vi "MTS_GenGridScanList.vi"(8 "Offsets":dbl[](array[numeric]), 9 "Points":u16[](array[numeric]), 11 "Starting":dbl[](array[numeric])) -> (0 "Grid Points":dbl[][](array[numeric]))   [LabVIEW 2011]
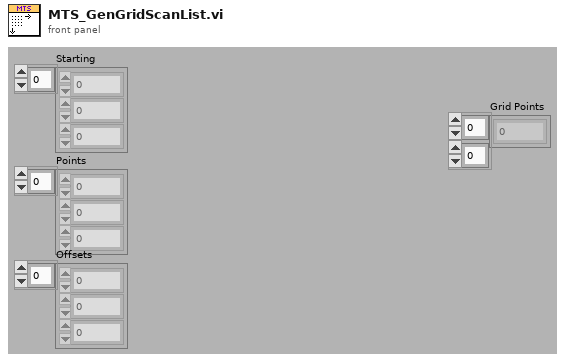
[diagram p1: front panel]
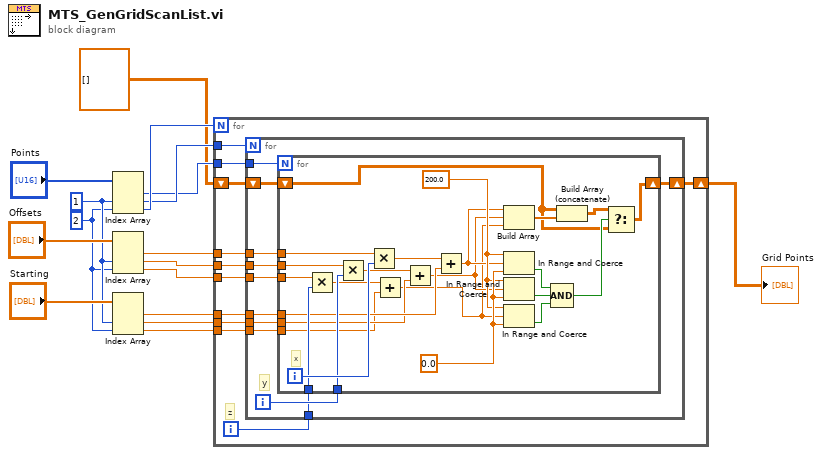
[diagram p0: block diagram]
diagram:
  w12 = 2 ("index")
  w13 = 1 ("index")
  n1 = Index Array(array="Points", index #2=w13, index #3=w12) -> (element #1=w9:u16, element #2=w10:u16, element #3=w11:u16)  [unwired: 1 in]
  n2 = Index Array(array="Offsets", index #2=w13, index #3=w12) -> (element #1=w5:dbl, element #2=w4:dbl, element #3=w3:dbl)  [unwired: 1 in]
  n3 = Index Array(array="Starting", index #2=w13, index #3=w12) -> (element #1=w8:dbl, element #2=w7:dbl, element #3=w6:dbl)  [unwired: 1 in]
  n4 = for {
    N: w11 -> [_]
    tunnel: w10 -> [w27]
    tunnel: w9 -> [w26]
    tunnel: w8 -> [w25]
    tunnel: w7 -> [w24]
    tunnel: w6 -> [w23]
    tunnel: w5 -> [w22]
    tunnel: w4 -> [w21]
    tunnel: w3 -> [w20]
    shift-right: [w17] -> w1
    shift-left: dbl[][] [] ("Grid Points") -> [w18]
    i -> [w19]
    # "z"
    n5 = for {
      N: w27 -> [_]
      tunnel: w26 -> [w38]
      tunnel: w25 -> [w37]
      tunnel: w24 -> [w36]
      tunnel: w23 -> [w35]
      tunnel: w22 -> [w34]
      tunnel: w21 -> [w33]
      tunnel: w20 -> [w32]
      tunnel: w19 -> [w30]
      shift-right: [w28] -> w17
      shift-left: w18 -> [w29]
      i -> [w31]
      # "y"
      n6 = for {
        N: w38 -> [_]
        tunnel: w37 -> [w54]
        tunnel: w36 -> [w53]
        tunnel: w35 -> [w52]
        tunnel: w34 -> [w63]
        tunnel: w33 -> [w62]
        tunnel: w32 -> [w61]
        tunnel: w31 -> [w59]
        tunnel: w30 -> [w58]
        shift-right: [w39] -> w28
        shift-left: w29 -> [w40]
        i -> [w60]
        w50 = 200.0 ("upper limit")
        w51 = 0.0 ("lower limit")
        # "x"
        n7 = Multiply(x=w61, y=w58) -> (x*y=w55:dbl)
        n8 = Multiply(x=w62, y=w59) -> (x*y=w56:dbl)
        n9 = Multiply(x=w63, y=w60) -> (x*y=w57:dbl)
        n10 = Add(x=w55, y=w52) -> (x+y=w44:dbl)
        n11 = Add(x=w56, y=w53) -> (x+y=w45:dbl)
        n12 = Add(x=w57, y=w54) -> (x+y=w46:dbl)
        n13 = Build Array(w46, w45, w44) -> (w43:dbl[])
        n14 = In Range and Coerce(upper limit=w50, x=w46, lower limit=w51) -> (In Range?=w49:bool)  [unwired: 1 out]
        n15 = In Range and Coerce(upper limit=w50, x=w45, lower limit=w51) -> (In Range?=w48:bool)  [unwired: 1 out]
        n16 = In Range and Coerce(upper limit=w50, x=w44, lower limit=w51) -> (In Range?=w47:bool)  [unwired: 1 out]
        n17 = Compound Arithmetic op=AND(w49, w48, w47) -> (w41:bool)
        n18 = Build Array (concatenate)(w40, w43) -> (w42:dbl[][])
        n19 = Select(t=w42, s=w41, f=w40) -> (s? t:f=w39:dbl[][])
      }
    }
  }
  "Grid Points" <- w1
